vi "Feedback.vi"(4 "TFF":dbl, 5 "x1_ref_norm_dot":dbl, 6 "a2":dbl, 7 "x2":dbl, 9 "a1":dbl, 10 "eHR":dbl, 11 "x1_norm":dbl) -> (2 "Vref":dbl, 3 "TM":dbl)   [LabVIEW 2013]
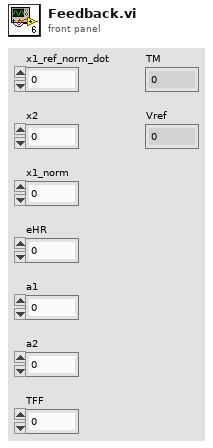
[diagram p1: front panel]
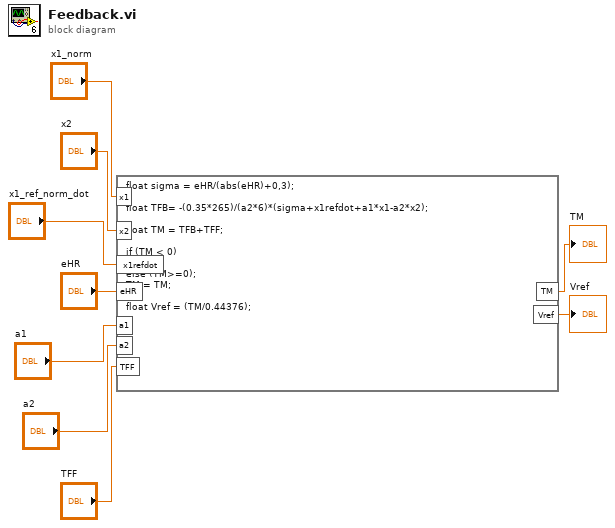
[diagram p0: block diagram]
diagram:
  n1 = formula code="float sigma = eHR/(abs(eHR)+0,3);\n\nfloat TFB= -(0.35*265)/(a2*6)*(sigma+x1refdot+a1*x1-a2*x2);\n\nfloat TM = TFB+TFF;\n\nif (TM < 0)\nTM = 0;\nelse (TM>=0);\nTM = TM;\n\nfloat Vref = (TM/0.44376);"("x1"="x1_norm", "x2"="x2", "x1refdot"="x1_ref_norm_dot", "eHR"="eHR", "a1"="a1", "a2"="a2", "TFF"="TFF") -> ("TM"=→"TM":dbl, "Vref"=→"Vref":dbl)
